vi "Draw Shapes.vi"(4 "Path Points":cluster{"x":dbl, "y":dbl}[](array[cluster]), 5 "Sample Period (s)":dbl=0.02, 6 "Output Point":T3, 7 "Commands":T2(array[cluster]) {"System Selection" items=["Elevator", "Floating Intake", "Carriage Intake"]; "System" items=["Elevator", "Floating Intake", "Carriage Intake"]}, 8 "Results":T4, 9 "new picture in":picture, 10 "Points":cluster{"x":dbl, "y":dbl, "th":dbl}[](array[cluster]), 11 "Picture in":refnum<vi>) -> (3 "new picture out":picture)   [LabVIEW 2018]
uses:
  2019 robot/Support Code/Availible Command systems for auto.ctl
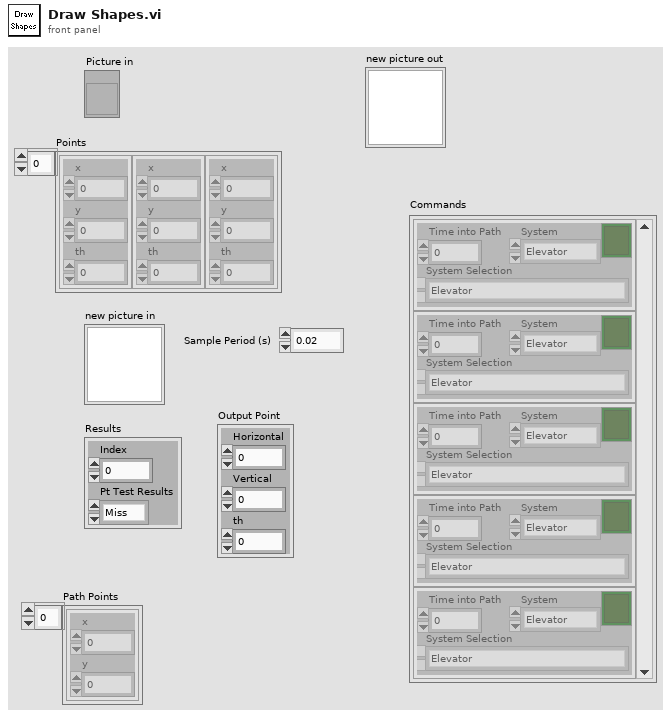
[diagram p1: front panel]
types:
  T1 = typedef "Availible Command systems for auto.ctl" = u16
  T2 = cluster{"Time into Path":dbl, "System":T1, "Item Selected?":bool, "System Selection":T1}[]
  T3 = cluster{"Horizontal":dbl, "Vertical":dbl, "th":dbl}
  T4 = cluster{"Index":i32, "Pt Test Results":enum16{"Miss", "Rect Hit", "Arrow Hit"}}
  T5 = cluster{i32, "Pt Test Results":enum16{"Miss", "Rect Hit", "Arrow Hit"}}
  T6 = typedef "LVPositionTypeDef.ctl" = cluster{"Left":i32, "Top":i32}
  T7 = typedef "LVBoundsTypeDef.ctl" = cluster{"Width":u32, "Height":u32}
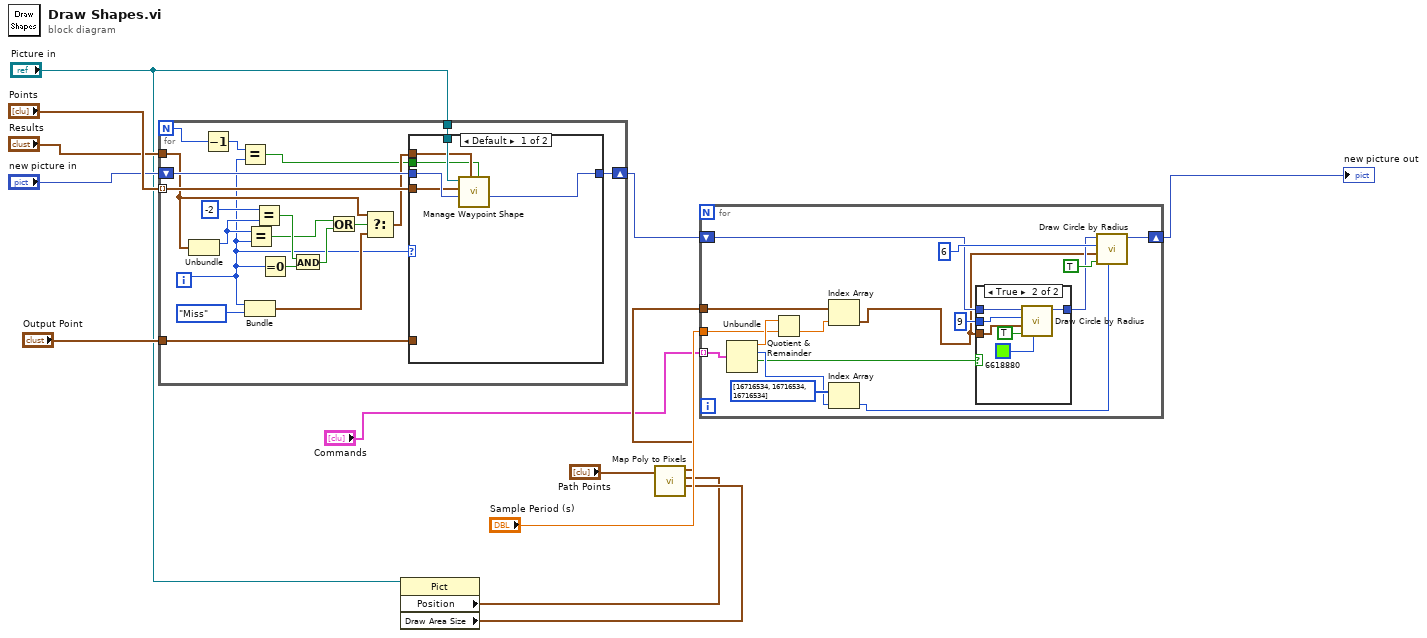
[diagram p0: block diagram]
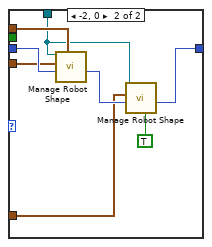
[diagram p3: hidden frame]
diagram:
  n1 = for {
    N -> [w18]
    tunnel: "Points" -> [w33] mode=indexing
    shift-right: [w32] -> w9
    shift-left: "new picture in" -> [w31]
    tunnel: "Picture in" -> [w30]
    tunnel: "Results" -> [w27]
    tunnel: "Output Point" -> [w14]
    i -> [w16]
    n2 = Unbundle(w27) -> ("Index"=w23:i32)  [unwired: 1 out]
    n3 = Decrement(x=w18) -> (x-1=w17:i32)
    n4 = Equal?(x=w17, y=w16) -> (x = y?=w15:bool)
    n5 = Bundle(w16, "Pt Test Results"=enum16{"Miss", "Rect Hit", "Arrow Hit"}."Miss") -> (w28:T5)  [unwired: 1 in]
    n6 = Equal?(x=w23, y=w16) -> (x = y?=w20:bool)
    n7 = Equal?(x=-2, y=w23) -> (x = y?=w22:bool)
    n8 = Equal To 0?(x=w16) -> (x = 0?=w25:bool)
    n9 = And(x=w22, y=w25) -> (x .and. y?=w21:bool)
    n10 = Or(x=w20, y=w21) -> (x .or. y?=w19:bool)
    n11 = Select(t=w27, s=w19, f=w28) -> (s? t:f=w29:T4)
    n12 = case shown="Default" w16 {
      tunnel: w33 -> [w35 w46]
      tunnel: [w38 w43] -> w32
      tunnel: w31 -> [w39 w47]
      tunnel: w30 -> [w37 w41]
      tunnel: w29 -> [w36 w45]
      tunnel: w15 -> [w34 _]
      tunnel: w14 -> [_ w42]
      frame Default {
        n13 = call "Manage Waypoint Shape.vi"("Draw Arrow"=w34, "Drawing Options"=w36, "new picture in"=w39, "Waypoint Position (ft)"=w35, "Pict Ref"=w37) -> ("new picture out"=w38:picture)  [unwired: 5 in, 1 out]
      }
      frame -2, 0 {
        n14 = call "Manage Robot Shape.vi"("Drawing Options"=w45, "new picture in"=w47, "Robot Position (ft)"=w46, "Pict Ref"=w41) -> ("new picture out"=w44:picture)  [unwired: 5 in, 2 out]
        n15 = call "Manage Robot Shape.vi"("Lighter"=TRUE ("Outline"), "new picture in"=w44, "Robot Position (ft)"=w42, "Pict Ref"=w41) -> ("new picture out"=w43:picture)  [unwired: 5 in, 2 out]
      }
    }
  }
  n16 = property on="Property Node" class="Pict"(reference="Picture in") -> ("Position"=w4:T6, "Draw Area Size"=w5:T7)  [unwired: 1 in, 2 out]
  n17 = call "Map Poly to Pixels.vi"("Draw Area Size"=w5, "Position"=w4, "Coords"="Path Points") -> ("Coords"=w2:cluster{"Horizontal":dbl, "Vertical":dbl}[])  [unwired: 8 in]
  n18 = for {
    shift-right: [w51] -> w8
    shift-left: w9 -> [w50]
    tunnel: "Commands" -> [w63] mode=indexing
    tunnel: w2 -> [w62]
    tunnel: "Sample Period (s)" -> [w60]
    n19 = Unbundle(w63) -> ("Time into Path"=w61:dbl, "System"=w57:T1, "Item Selected?"=w53:bool)  [unwired: 1 out]
    n20 = Quotient & Remainder(x=w61, y=w60) -> (floor(x/y)=w59:dbl)  [unwired: 1 out]
    n21 = Index Array(array=w62, index=w59) -> (element=w48:cluster{"Horizontal":dbl, "Vertical":dbl})
    n22 = Index Array(array=u32[] [16716534, 16716534, 16716534], index=w57) -> (element=w56:u32)
    n23 = case shown="True" w53 {
      tunnel: [w64 w69] -> w52
      tunnel: w50 -> [w64 w70]
      tunnel: i16 9 ("radius") -> [_ w68]
      tunnel: w48 -> [_ w66]
      frame False {
      }
      frame True {
        n24 = call <vilib>:"Draw Circle by Radius.vi"("color(black)"=u32 6618880, "fill?(F)"=TRUE, "pixel center"=w66, "radius"=w68, "picture"=w70) -> ("new picture"=w69:picture)  [unwired: 6 in]
      }
    }
    n25 = call <vilib>:"Draw Circle by Radius.vi"("color(black)"=w56, "fill?(F)"=TRUE, "pixel center"=w48, "radius"=i16 6, "picture"=w52) -> ("new picture"=w51:picture)  [unwired: 6 in]
  }
  "new picture out" <- w8
